vi "Release Semaphore (Even if Error).vi"(8 "error in (no error)":errorcluster, 11 "semaphore":T1) -> (0 "error out":errorcluster, 3 "semaphore out":T1)   [LabVIEW 2020, in "JKI TCP Server.lvclass"]
uses:
  JKI TCP Server.lvclass
panel:
  # "Copyright © 2006 James Kring, Inc. All rights reserved.\n\nAuthor: Philippe Guerit <philippe.guerit@jameskring.com>\n<alternate_email: PJM_LabVIEW@yahoo.com>\n\nThis library is provided \"AS IS\" , WITHOUT WARRANTIES OR \nCONDITIONS OF ANY KIND, either express or implied.\n\nJames Kring, Inc. -- http://www.jameskring.com"
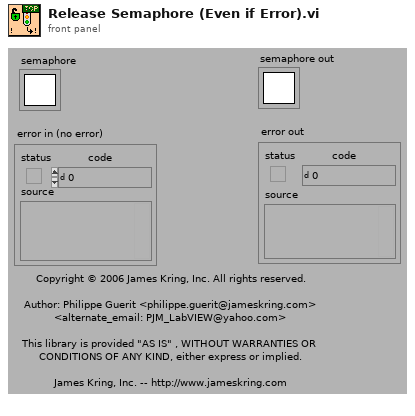
[diagram p1: front panel]
types:
  T1 = typedef "Semaphore RefNum" = refnum<k1>
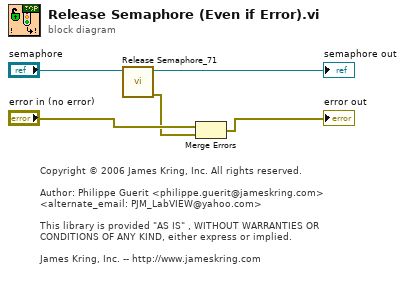
[diagram p0: block diagram]
diagram:
  # "Copyright © 2006 James Kring, Inc. All rights reserved.\n\nAuthor: Philippe Guerit <philippe.guerit@jameskring.com>\n<alternate_email: PJM_LabVIEW@yahoo.com>\n\nThis library is provided \"AS IS\" , WITHOUT WARRANTIES OR \nCONDITIONS OF ANY KIND, either express or implied.\n\nJames Kring, Inc. -- http://www.jameskring.com"
  n1 = call <vilib>:"Release Semaphore_71.vi"("semaphore"="semaphore") -> ("error out"=w1:errorcluster, "semaphore out"=→"semaphore out":T1)  [unwired: 5 in]
  n2 = Merge Errors("error in (no error)", w1) -> (→"error out":errorcluster)
